vi "Measurement Logic.vi"(8 "error in":errorcluster, 11 "Measurement Configuration":T2) -> (0 "error out":errorcluster, 3 "Measurement Results":T1 {"Load Regulation (mV/mA)" format="%#.5g"})   [LabVIEW 2020, in "Load Regulation.lvlib"]
uses:
  Load Regulation.lvlib
  Reusables/Stimulus And Measure.ctl
  Reusables/Load Output Function.ctl
  Reusables/Prepare Fn Configurations.ctl
  Reusables/Advanced Settings.ctl
  26cf059d-6099-420a-9488-44e269848c92.vi
  TestResults.ctl
  TestInputs.ctl
  Measurement Results.ctl
  Measurement Configuration.ctl
panel:
  out "Load Regulation":cluster{"Iload (mA)":dbl[], "Vout (V)":dbl[]}(graph)
  out "Load Regulation (%)":dbl format="%#.3g"
  out "Load Regulation (mV/mA)":dbl format="%#.3g"
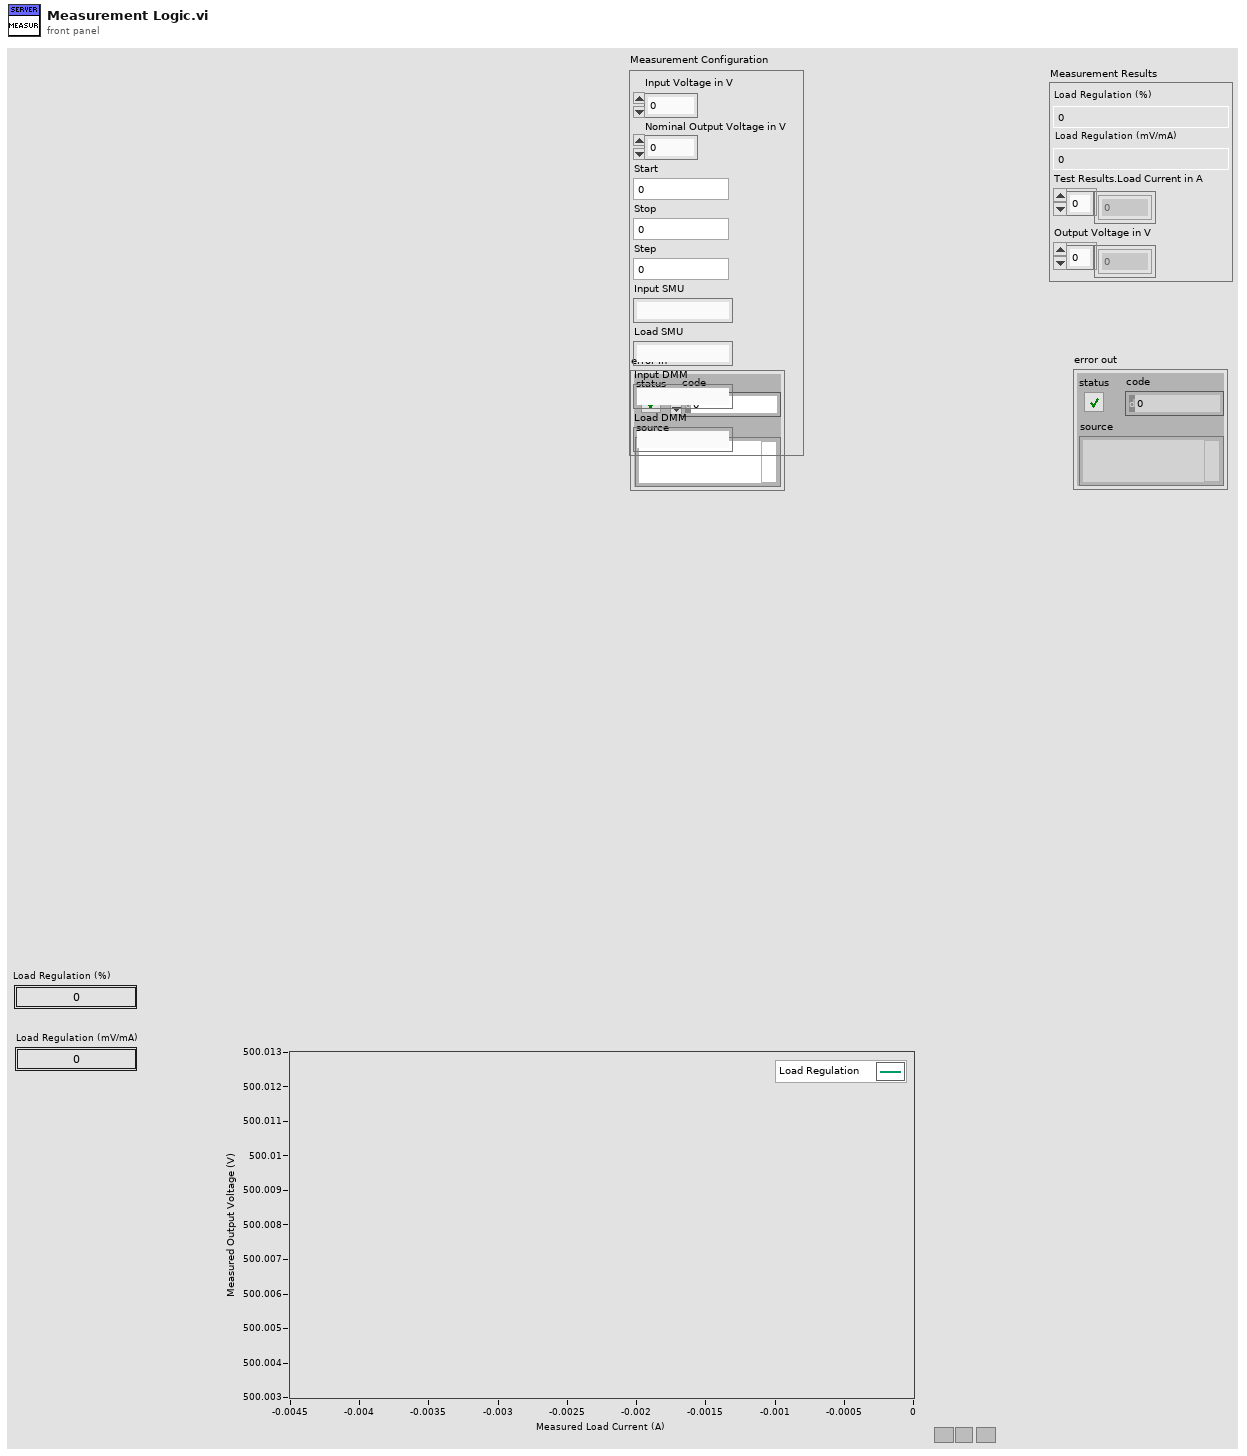
[diagram p1: front panel]
types:
  T1 = typedef "Load Regulation.lvlib/Measurement Results.ctl" = cluster{"Load Regulation (%)":dbl, "Load Regulation (mV/mA)":dbl, "Test Results.Load Current in A":dbl[], "Output Voltage in V":dbl[]}
  T2 = typedef "Load Regulation.lvlib/Measurement Configuration.ctl" = cluster{"Input Voltage in V":dbl, "Nominal Output Voltage in V":dbl, "Start":dbl, "Stop":dbl, "Step":dbl, "Input SMU":string, "Load SMU":string, "Input DMM":string, "Load DMM":string}
  T3 = typedef "Load Regulation.lvlib/TestInputs.ctl" = cluster{"Input Voltage in V":dbl, "Load Current in A":dbl[], "Nominal Output Voltage in V":dbl, "Advance Setting":T4}
  T4 = typedef "Advanced Settings.ctl" = cluster{"Prepare":T5, "Stimulus And Measure":T7}
  T5 = typedef "Prepare Fn Configurations.ctl" = cluster{"Load SMU Output Function":T6}
  T6 = typedef "Load Output Function.ctl" = enum16{"VoltageSource", "CurrentSource"}
  T7 = typedef "Stimulus And Measure.ctl" = cluster{"Loop Delay in milliSecond":u32}
  T8 = typedef "Load Regulation.lvlib/TestResults.ctl" = cluster{"Input Voltage in V":dbl[], "Input Current in A":dbl[], "Output Voltage in V":dbl[], "Load Current in A":dbl[], "Load Regulation in mV/mA":dbl, "Load Regulation in %":dbl}
  T9 = cluster{"Test Inputs":T3, "Test Results":T8, "Test Results[][]":string[][], "Input SMU":refnum<k15>, "Input DMM":refnum<k15>, "Load DMM":refnum<k15>, "Load SMU":refnum<k15>}
  T10 = cluster{"Load Current in A":dbl[], "Output Voltage in V":dbl[]}
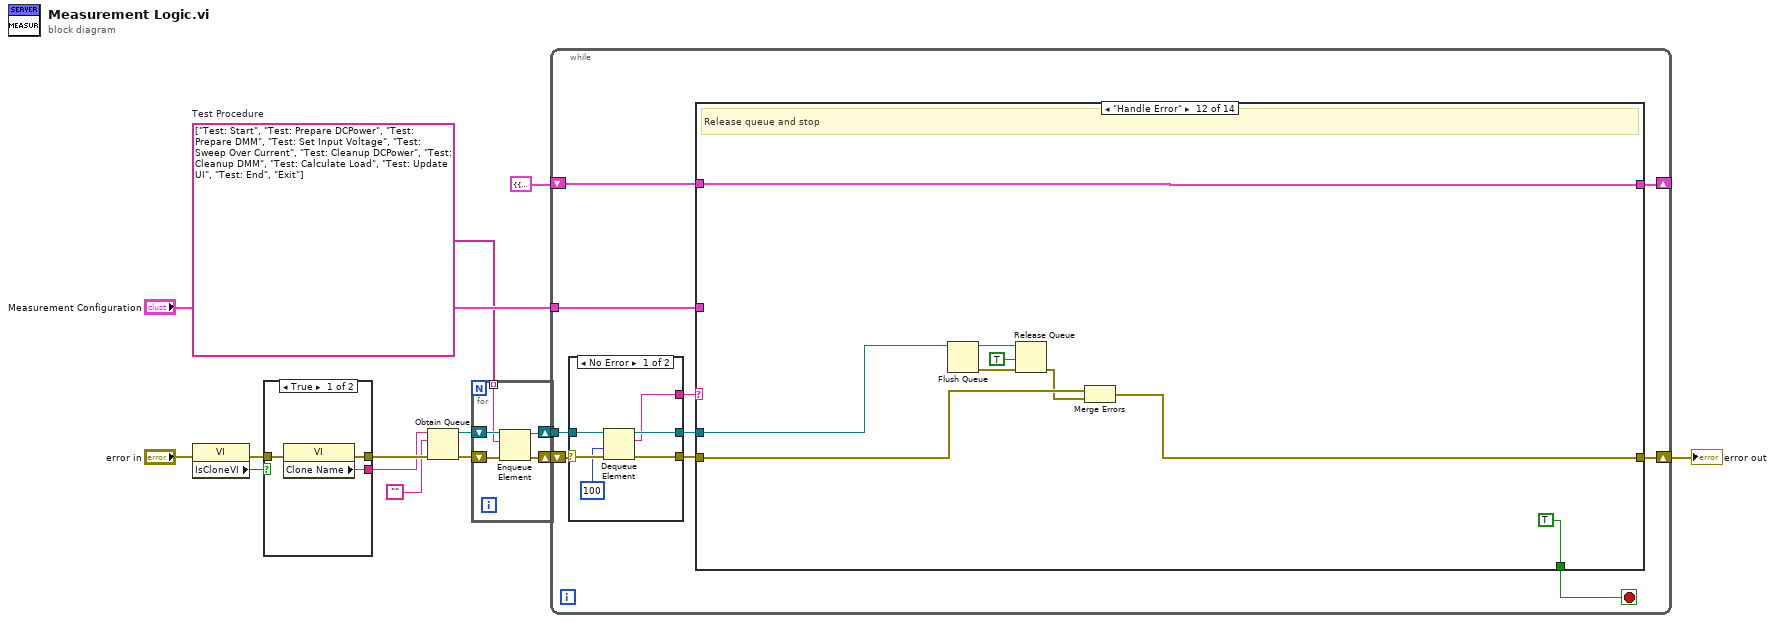
[diagram p0: block diagram]
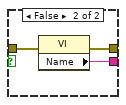
[diagram p2: hidden frame]
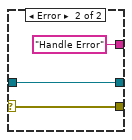
[diagram p3: hidden frame]
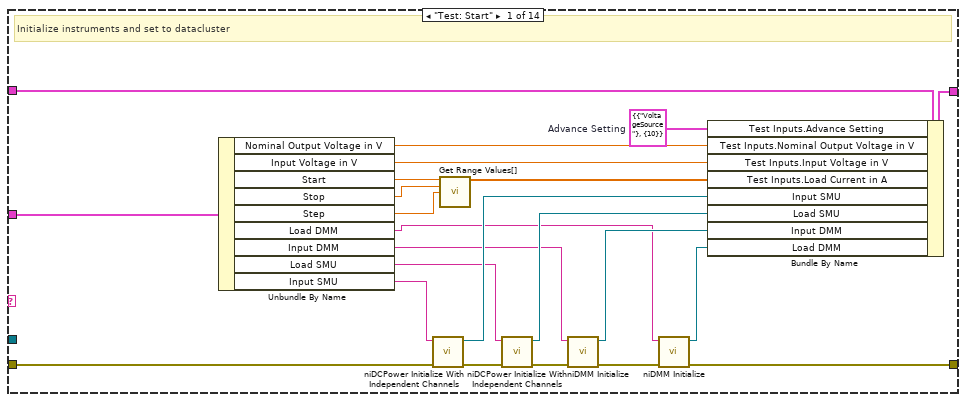
[diagram p4: hidden frame]
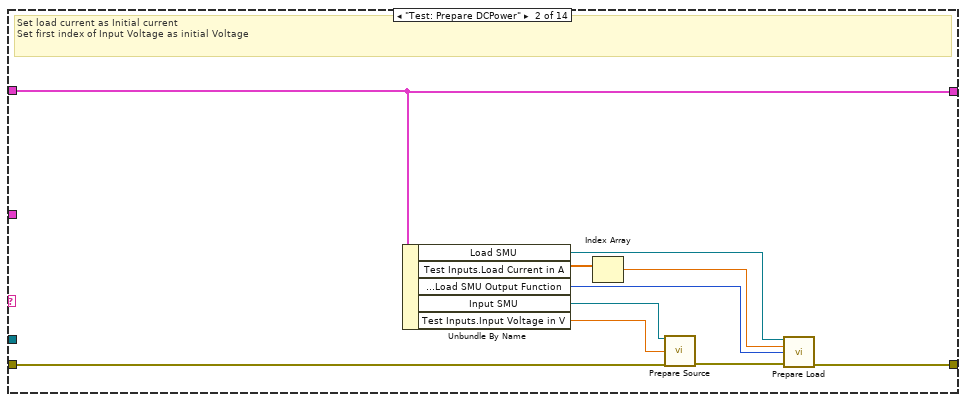
[diagram p5: hidden frame]
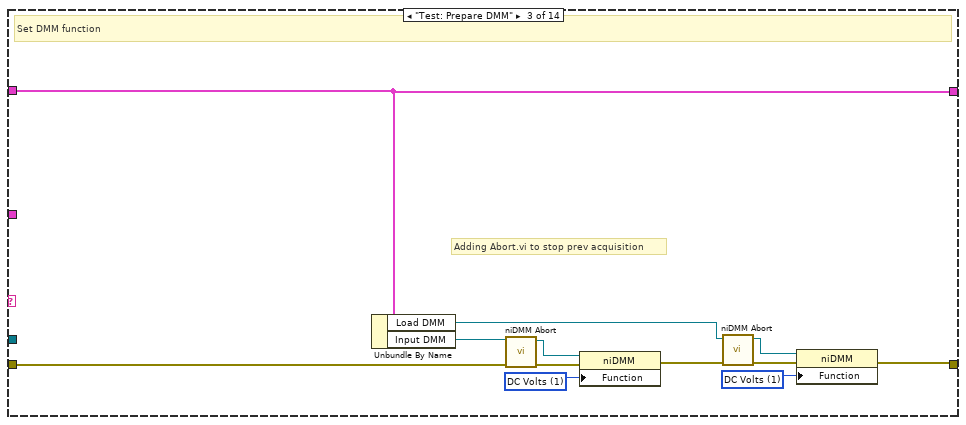
[diagram p6: hidden frame]
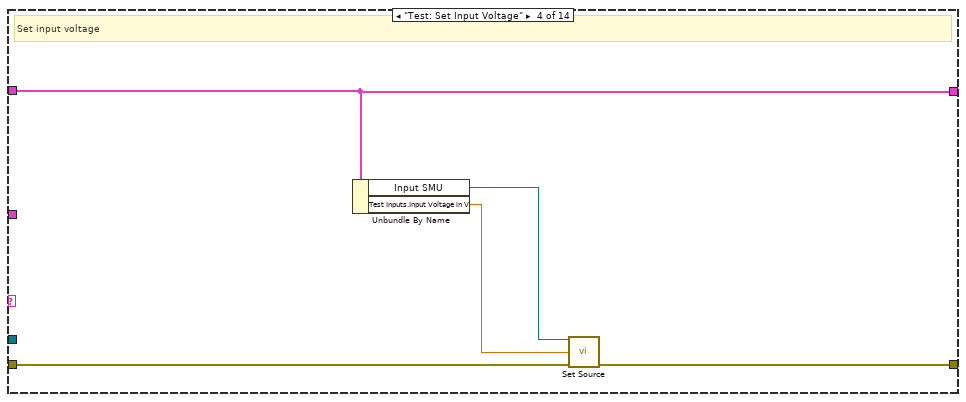
[diagram p7: hidden frame]
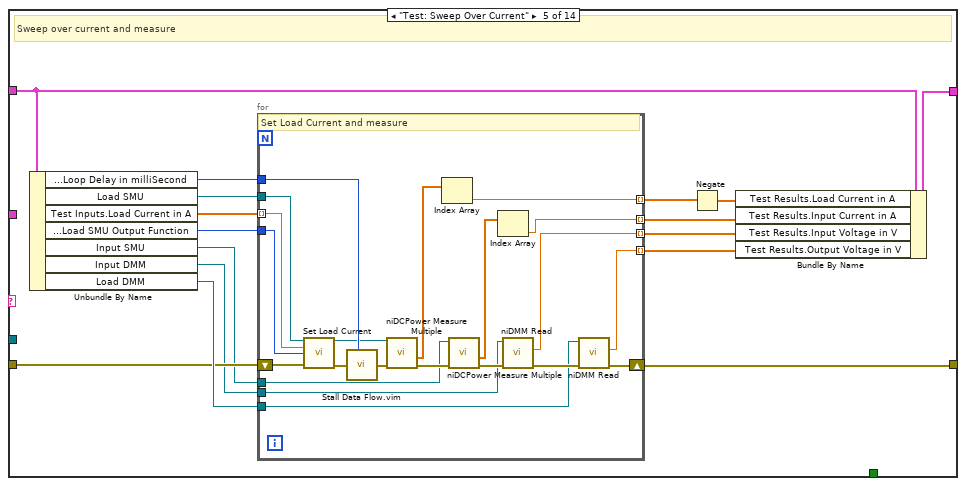
[diagram p8: hidden frame]
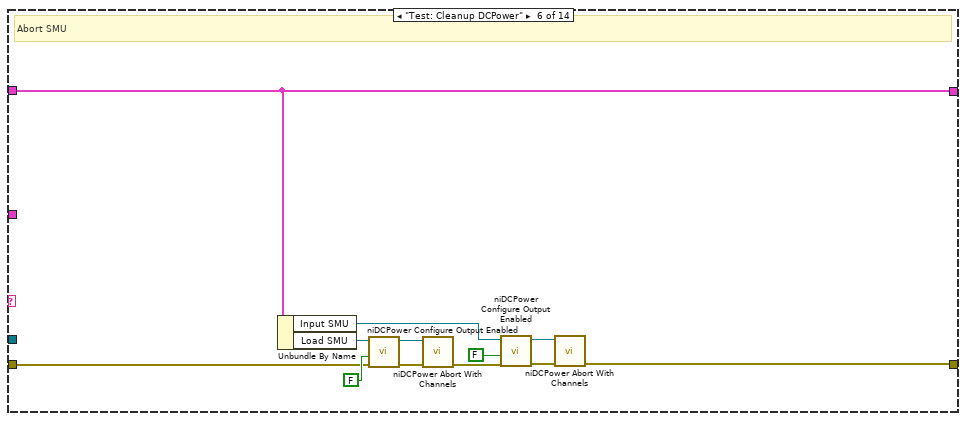
[diagram p9: hidden frame]
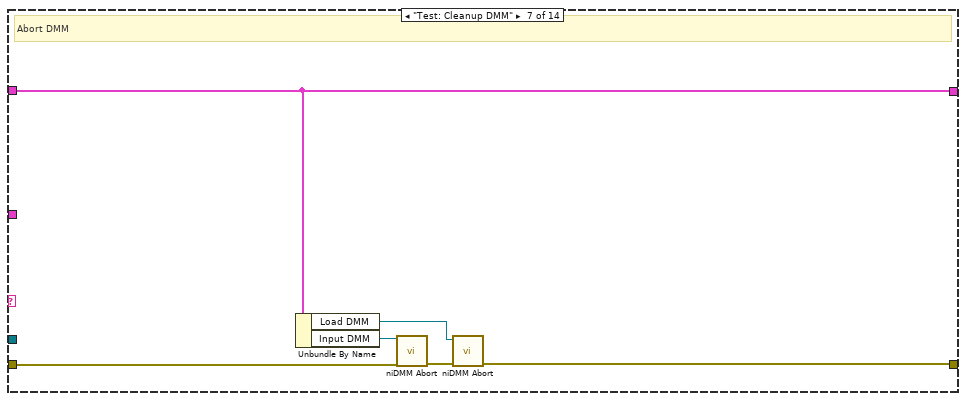
[diagram p10: hidden frame]
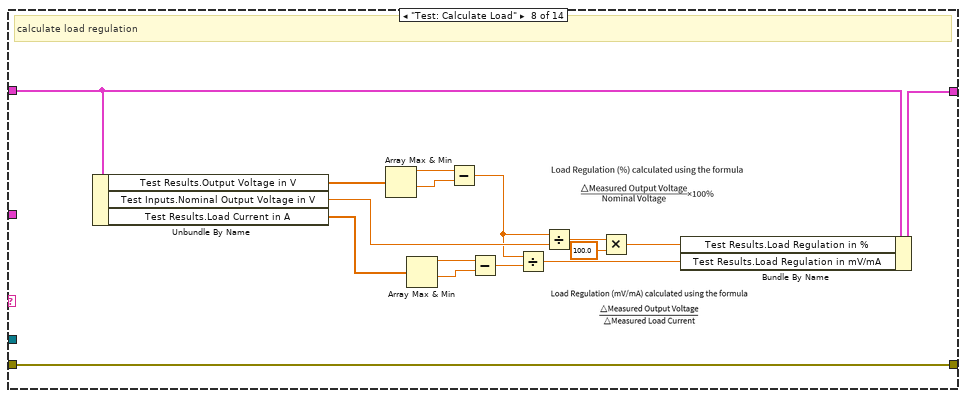
[diagram p11: hidden frame]
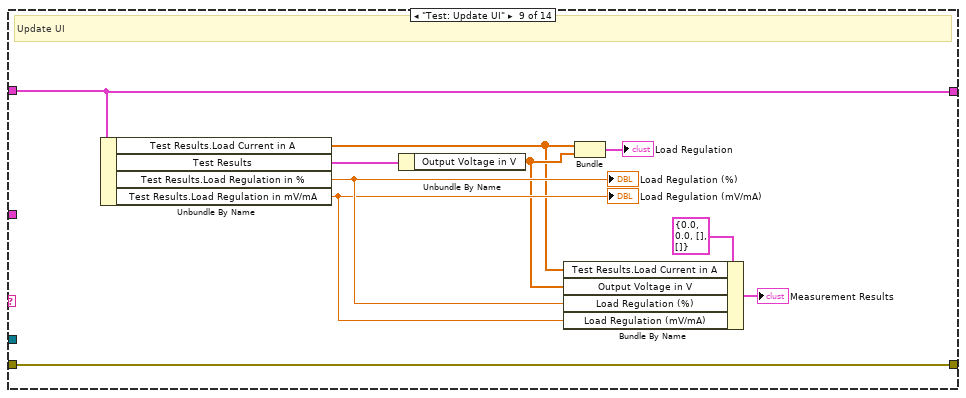
[diagram p12: hidden frame]
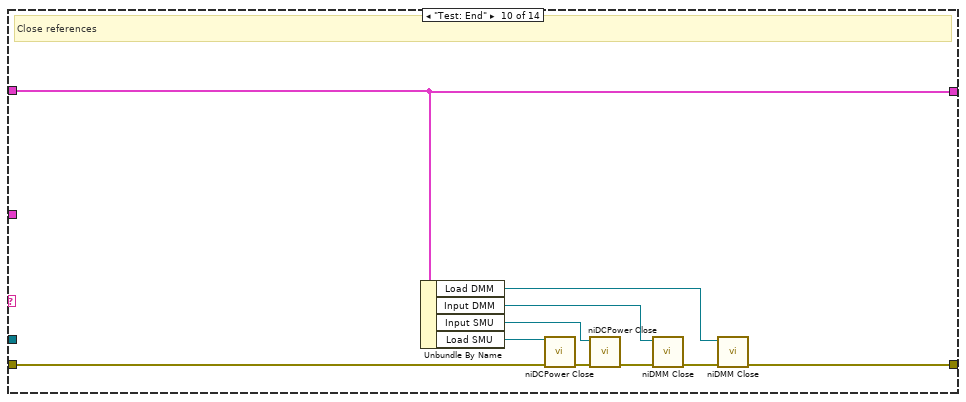
[diagram p13: hidden frame]
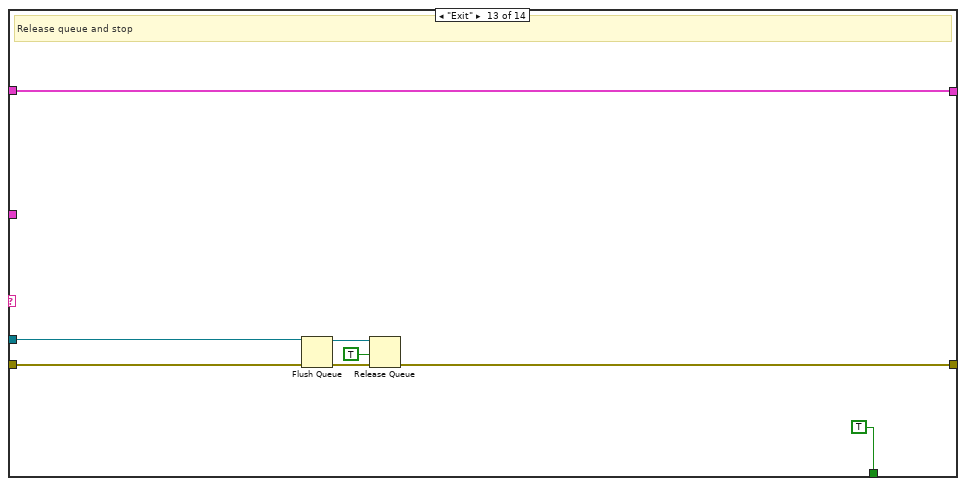
[diagram p15: hidden frame]
diagram:
  w2 = string[] ["Test: Start", "Test: Prepare DCPower", "Test: Prepare DMM", "Test: Set Input Voltage", "Test: Sweep Over Current", "Test: Cleanup DCPower", "Test: Cleanup DMM", "Test: Calculate Load", "Test: Update UI", "Test: End", "Exit"]  # Test Procedure
  n1 = property class="VI"(error in="error in") -> (error out=w7:errorcluster, "IsCloneVI"=w8:bool)  [unwired: 1 in, 1 out]
  n2 = case shown="True" w8 {
    tunnel: [w17 w20] -> w13
    tunnel: [w16 w19] -> w12
    tunnel: w7 -> [w15 w18]
    frame True {
      n3 = property class="VI"(error in=w15) -> (error out=w17:errorcluster, "Clone Name"=w16:string)  [unwired: 1 in, 1 out]
    }
    frame False {
      n4 = property class="VI"(error in=w18) -> (error out=w20:errorcluster, "Name"=w19:string)  [unwired: 1 in, 1 out]
    }
  }
  n5 = Obtain Queue(name (unnamed)=w12, element data type="", error in (no error)=w13) -> (queue out=w10:refnum<queue>, error out=w11:errorcluster)  [unwired: 2 in, 1 out]
  n6 = for {
    shift-right: [w22] -> w5
    shift-left: w11 -> [w25]
    shift-right: [w23] -> w6
    shift-left: w10 -> [w24]
    tunnel: w2 -> [w21] mode=indexing
    n7 = Enqueue Element(queue=w24, element=w21, error in (no error)=w25) -> (queue out=w23:refnum<queue>, error out=w22:errorcluster)  [unwired: 1 in, 1 out]
  }
  n8 = while {
    tunnel: w6 -> [w30]
    shift-right: [w35] -> w1
    shift-left: w5 -> [w31]
    shift-right: [w33] -> _
    shift-left: T9 {"Test Inputs"={"Input Voltage in V"=0.0, "Load Current in A"=[], "Nominal Output Voltage in V"=0.0, "Advance Setting"={"Prepare"={"Load SMU Output Function"=enum."VoltageSource"}, "Stimulus And Measure"={"Loop Delay in milliSecond"=1}}}, "Test Results"={"Input Voltage in V"=[], "Input Current in A"=[], "Output Voltage in V"=[], "Load Current in A"=[], "Load Regulation in mV/mA"=0.0, "Load Regulation in %"=0.0}, "Test Results[][]"=[], "Input SMU"="", "Input DMM"="", "Load DMM"="", "Load SMU"=""} -> [w34]
    tunnel: "Measurement Configuration" -> [w26]
    stop <- w32 stop-if-true
    n9 = case shown="No Error" w31 {
      selector: w31 -> [w41 w44]
      tunnel: [w40 w44] -> w27
      tunnel: w30 -> [w39 w43]
      tunnel: [w38 w43] -> w28
      tunnel: [w37 "Handle Error"] -> w29
      frame No Error {
        n10 = Dequeue Element(queue=w39, timeout in ms (-1)=100, error in (no error)=w41) -> (queue out=w38:refnum<queue>, element=w37:string, error out=w40:errorcluster)  [unwired: 1 out]
      }
      frame Error {
      }
    }
    n11 = case shown="\"Handle Error\"" w29 {
      tunnel: w28 -> [_ _ _ _ _ _ _ _ _ _ _ w188 w197 _]
      tunnel: w27 -> [w49 w70 w78 w90 w99 w132 w144 w150 w168 w176 w187 w194 w199 w205]
      tunnel: [w62 w71 w80 w91 w102 w140 w147 w150 w168 w179 w187 w195 w198 w205] -> w35
      tunnel: w34 -> [w66 w76 w86 w94 w100 w139 w149 w151 w173 w185 w186 w196 w204 w206]
      tunnel: [w67 w76 w86 w94 w101 w139 w149 w152 w173 w185 w186 w196 w204 w206] -> w33
      tunnel: [_ _ _ _ _ _ _ _ _ _ _ TRUE TRUE _] -> w32
      tunnel: w26 -> [w45 _ _ _ _ _ _ _ _ _ _ _ _ _]
      frame "Test: Start" {
        w48 = T4 {"Prepare"={"Load SMU Output Function"=enum."VoltageSource"}, "Stimulus And Measure"={"Loop Delay in milliSecond"=10}}  # Advance Setting
        # "Initialize instruments and set to datacluster"
        n12 = Unbundle By Name(w45) -> ("Nominal Output Voltage in V"=w57:dbl, "Input Voltage in V"=w46:dbl, "Start"=w56:dbl, "Stop"=w55:dbl, "Step"=w54:dbl, "Load DMM"=w50:string, "Input DMM"=w51:string, "Load SMU"=w52:string, "Input SMU"=w53:string)
        n13 = call <instrlib>:"niDCPower Initialize With Independent Channels.vi"("error in (no error)"=w49, "resource name"=w53) -> ("error out"=w61:errorcluster, "instrument handle out"=w65:refnum<k15>)  [unwired: 8 in]
        n14 = call "Get Range Values[].vi"("Start"=w56, "Stop"=w55, "Step Size"=w54) -> ("Values[]"=w47:dbl[])  [unwired: 12 in]
        n15 = call <instrlib>:"niDCPower Initialize With Independent Channels.vi"("error in (no error)"=w61, "resource name"=w52) -> ("error out"=w60:errorcluster, "instrument handle out"=w58:refnum<k15>)  [unwired: 8 in]
        n16 = call <instrlib>:"niDMM Initialize.vi"("error in (no error)"=w60, "Instrument Descriptor"=w51) -> ("error out"=w63:errorcluster, "instrument handle out"=w59:refnum<k15>)  [unwired: 8 in]
        n17 = call <instrlib>:"niDMM Initialize.vi"("error in (no error)"=w63, "Instrument Descriptor"=w50) -> ("error out"=w62:errorcluster, "instrument handle out"=w64:refnum<k15>)  [unwired: 8 in]
        n18 = Bundle By Name(cluster=w66, "Test Inputs.Advance Setting"=w48, "Test Inputs.Nominal Output Voltage in V"=w57, "Test Inputs.Input Voltage in V"=w46, "Test Inputs.Load Current in A"=w47, "Input SMU"=w65, "Load SMU"=w58, "Input DMM"=w59, "Load DMM"=w64) -> (w67:T9)
      }
      frame "Test: Prepare DCPower" {
        # "Set load current as Initial current\nSet first index of Input Voltage as initial Voltage"
        n19 = Unbundle By Name(w76) -> ("Load SMU"=w74:refnum<k15>, "Test Inputs.Load Current in A"=w73:dbl[], "Test Inputs.Advance Setting.Prepare.Load SMU Output Function"=w68:T6, "Input SMU"=w75:refnum<k15>, "Test Inputs.Input Voltage in V"=w77:dbl)
        n20 = Index Array(array=w73) -> (element=w69:dbl)  [unwired: 1 in]
        n21 = call "Prepare Source.vi"("instrument handle"=w75, "Initial Voltage Level (V)"=w77, "error in (no error)"=w70) -> ("error out"=w72:errorcluster)  [unwired: 12 in]
        n22 = call "Prepare Load.vi"("instrument handle"=w74, "Load Current Level (A)"=w69, "Load Output Function"=w68, "error in (no error)"=w72) -> ("error out"=w71:errorcluster)  [unwired: 11 in]
      }
      frame "Test: Prepare DMM" {
        w82 = 1 items=["DC Volts"=1, "AC Volts"=2, "DC Current"=3, "AC Current"=4, "2-Wire Resistance"=5, "4-Wire Resistance"=101, "Frequency"=104, "Period"=105, "AC Volts DC Coupled"=1001, "Diode"=1002, "Waveform Voltage"=1003, "Waveform Current"=1004, "Capacitance"=1005, "Inductance"=1006, "Temperature"=108] ("Configuration:Function")
        w89 = 1 items=["DC Volts"=1, "AC Volts"=2, "DC Current"=3, "AC Current"=4, "2-Wire Resistance"=5, "4-Wire Resistance"=101, "Frequency"=104, "Period"=105, "AC Volts DC Coupled"=1001, "Diode"=1002, "Waveform Voltage"=1003, "Waveform Current"=1004, "Capacitance"=1005, "Inductance"=1006, "Temperature"=108] ("Configuration:Function")
        # "Adding Abort.vi to stop prev acquisition"
        # "Set DMM function"
        n23 = Unbundle By Name(w86) -> ("Load DMM"=w79:refnum<k15>, "Input DMM"=w85:refnum<k15>)
        n24 = call <instrlib>:"niDMM Abort.vi"("error in (no error)"=w78, "instrument handle"=w85) -> ("error out"=w88:errorcluster, "instrument handle out"=w87:refnum<k15>)  [unwired: 8 in]
        n25 = property class="niDMM"(reference=w87, error in=w88, "Function"=w89) -> (error out=w81:errorcluster)  [unwired: 1 out]
        n26 = call <instrlib>:"niDMM Abort.vi"("error in (no error)"=w81, "instrument handle"=w79) -> ("error out"=w83:errorcluster, "instrument handle out"=w84:refnum<k15>)  [unwired: 8 in]
        n27 = property class="niDMM"(reference=w84, error in=w83, "Function"=w82) -> (error out=w80:errorcluster)  [unwired: 1 out]
      }
      frame "Test: Set Input Voltage" {
        # "Set input voltage"
        n28 = Unbundle By Name(w94) -> ("Input SMU"=w93:refnum<k15>, "Test Inputs.Input Voltage in V"=w92:dbl)
        n29 = call "Set Source.vi"("instrument handle in"=w93, "Vin in V"=w92, "error in (no error)"=w90) -> ("error out"=w91:errorcluster)  [unwired: 11 in, 1 out]
      }
      frame "Test: Sweep Over Current" {
        # "Sweep over current and measure"
        n30 = Unbundle By Name(w100) -> ("Test Inputs.Advance Setting.Stimulus And Measure.Loop Delay in milliSecond"=w108:u32, "Load SMU"=w110:refnum<k15>, "Test Inputs.Load Current in A"=w109:dbl[], "Test Inputs.Advance Setting.Prepare.Load SMU Output Function"=w98:T6, "Input SMU"=w95:refnum<k15>, "Input DMM"=w96:refnum<k15>, "Load DMM"=w107:refnum<k15>)
        n31 = for {
          tunnel: w110 -> [w130]
          tunnel: w109 -> [w113] mode=indexing
          tunnel: w108 -> [w128]
          tunnel: w96 -> [w121]
          tunnel: w107 -> [w120]
          tunnel: [w114] -> w106 mode=indexing
          tunnel: [w115] -> w105 mode=indexing
          tunnel: [w119] -> w104 mode=indexing
          tunnel: [w118] -> w103 mode=indexing
          shift-right: [w117] -> w102
          shift-left: w99 -> [w131]
          tunnel: w98 -> [w112]
          tunnel: w95 -> [w111]
          # "Set Load Current and measure"
          n32 = call "Set Load Current.vi"("instrument handle in"=w130, "current level"=w113, "OutputFunction"=w112, "error in (no error)"=w131) -> ("instrument handle out"=w116:refnum<k15>, "error out"=w129:errorcluster)  [unwired: 10 in]
          n33 = call "Stall Data Flow.vim"("value in"=w129, "milliseconds to wait"=w128) -> ("value out"=w122:errorcluster)  [unwired: 1 out]
          n34 = call <instrlib>:"niDCPower Measure Multiple.vi"("error in (no error)"=w122, "instrument handle"=w116) -> ("error out"=w124:errorcluster, "current measurements"=w127:dbl[])  [unwired: 6 in, 2 out]
          n35 = Index Array(array=w127) -> (element=w115:dbl)  [unwired: 1 in]
          n36 = call <instrlib>:"niDCPower Measure Multiple.vi"("error in (no error)"=w124, "instrument handle"=w111) -> ("error out"=w123:errorcluster, "current measurements"=w125:dbl[])  [unwired: 6 in, 2 out]
          n37 = Index Array(array=w125) -> (element=w114:dbl)  [unwired: 1 in]
          n38 = call <instrlib>:"niDMM Read.vi"("error in (no error)"=w123, "instrument handle"=w121) -> ("error out"=w126:errorcluster, "Measurement"=w119:dbl)  [unwired: 7 in, 1 out]
          n39 = call <instrlib>:"niDMM Read.vi"("error in (no error)"=w126, "instrument handle"=w120) -> ("error out"=w117:errorcluster, "Measurement"=w118:dbl)  [unwired: 7 in, 1 out]
        }
        n40 = Negate(x=w105) -> (-x=w97:dbl[])
        n41 = Bundle By Name(cluster=w100, "Test Results.Load Current in A"=w97, "Test Results.Input Current in A"=w106, "Test Results.Input Voltage in V"=w104, "Test Results.Output Voltage in V"=w103) -> (w101:T9)
      }
      frame "Test: Cleanup DCPower" {
        # "Abort SMU"
        n42 = Unbundle By Name(w139) -> ("Input SMU"=w138:refnum<k15>, "Load SMU"=w133:refnum<k15>)
        n43 = call <instrlib>:"niDCPower Configure Output Enabled.vi"("error in (no error)"=w132, "output enabled"=FALSE, "instrument handle"=w133) -> ("error out"=w134:errorcluster, "instrument handle out"=w137:refnum<k15>)  [unwired: 7 in]
        n44 = call <instrlib>:"niDCPower Abort With Channels.vi"("error in (no error)"=w134, "instrument handle"=w137) -> ("error out"=w135:errorcluster)  [unwired: 8 in, 1 out]
        n45 = call <instrlib>:"niDCPower Configure Output Enabled.vi"("error in (no error)"=w135, "output enabled"=FALSE, "instrument handle"=w138) -> ("error out"=w142:errorcluster, "instrument handle out"=w141:refnum<k15>)  [unwired: 7 in]
        n46 = call <instrlib>:"niDCPower Abort With Channels.vi"("error in (no error)"=w142, "instrument handle"=w141) -> ("error out"=w140:errorcluster)  [unwired: 8 in, 1 out]
      }
      frame "Test: Cleanup DMM" {
        # "Abort DMM"
        n47 = Unbundle By Name(w149) -> ("Load DMM"=w146:refnum<k15>, "Input DMM"=w145:refnum<k15>)
        n48 = call <instrlib>:"niDMM Abort.vi"("error in (no error)"=w144, "instrument handle"=w145) -> ("error out"=w148:errorcluster)  [unwired: 8 in, 1 out]
        n49 = call <instrlib>:"niDMM Abort.vi"("error in (no error)"=w148, "instrument handle"=w146) -> ("error out"=w147:errorcluster)  [unwired: 8 in, 1 out]
      }
      frame "Test: Calculate Load" {
        # "calculate load regulation"
        n50 = Unbundle By Name(w151) -> ("Test Results.Output Voltage in V"=w162:dbl[], "Test Inputs.Nominal Output Voltage in V"=w160:dbl, "Test Results.Load Current in A"=w157:dbl[])
        n51 = Array Max & Min(array=w162) -> (max value=w165:dbl, min value=w161:dbl)  [unwired: 2 out]
        n52 = Array Max & Min(array=w157) -> (max value=w158:dbl, min value=w159:dbl)  [unwired: 2 out]
        n53 = Subtract(x=w165, y=w161) -> (x-y=w156:dbl)
        n54 = Subtract(x=w158, y=w159) -> (x-y=w155:dbl)
        n55 = Divide(x=w156, y=w155) -> (x/y=w154:dbl)
        n56 = Divide(x=w156, y=w160) -> (x/y=w164:dbl)
        n57 = Multiply(x=w164, y=100.0) -> (x*y=w163:dbl)
        n58 = Bundle By Name(cluster=w151, "Test Results.Load Regulation in %"=w163, "Test Results.Load Regulation in mV/mA"=w154) -> (w152:T9)
      }
      frame "Test: Update UI" {
        # "Update UI"
        n59 = Unbundle By Name(w173) -> ("Test Results.Load Current in A"=w169:dbl[], "Test Results"=w175:T8, "Test Results.Load Regulation in %"=w172:dbl, "Test Results.Load Regulation in mV/mA"=w171:dbl)
        "Load Regulation (%)" <- w172
        "Load Regulation (mV/mA)" <- w171
        n60 = Unbundle By Name(w175) -> ("Output Voltage in V"=w170:dbl[])
        n61 = Bundle By Name(cluster=T1 {"Load Regulation (%)"=0.0, "Load Regulation (mV/mA)"=0.0, "Test Results.Load Current in A"=[], "Output Voltage in V"=[]} ("Measurement Results"), "Test Results.Load Current in A"=w169, "Output Voltage in V"=w170, "Load Regulation (%)"=w172, "Load Regulation (mV/mA)"=w171) -> (→"Measurement Results":T1)
        n62 = Bundle("Load Current in A"=w169, "Output Voltage in V"=w170) -> (→"Load Regulation":T10)  [unwired: 1 in]
      }
      frame "Test: End" {
        # "Close references"
        n63 = Unbundle By Name(w185) -> ("Load DMM"=w180:refnum<k15>, "Input DMM"=w181:refnum<k15>, "Input SMU"=w184:refnum<k15>, "Load SMU"=w178:refnum<k15>)
        n64 = call <instrlib>:"niDCPower Close.vi"("error in (no error)"=w176, "instrument handle"=w178) -> ("error out"=w177:errorcluster)  [unwired: 9 in]
        n65 = call <instrlib>:"niDCPower Close.vi"("error in (no error)"=w177, "instrument handle"=w184) -> ("error out"=w183:errorcluster)  [unwired: 9 in]
        n66 = call <instrlib>:"niDMM Close.vi"("error in (no error)"=w183, "instrument handle"=w181) -> ("error out"=w182:errorcluster)  [unwired: 9 in]
        n67 = call <instrlib>:"niDMM Close.vi"("error in (no error)"=w182, "instrument handle"=w180) -> ("error out"=w179:errorcluster)  [unwired: 9 in]
      }
      frame "----Misc------" {
      }
      frame "Handle Error" {
        # "Release queue and stop"
        n68 = Flush Queue(queue=w188) -> (queue out=w192:refnum<queue>, error out=w191:errorcluster)  [unwired: 1 in, 1 out]
        n69 = Release Queue(queue=w192, force destroy? (F)=TRUE, error in (no error)=w191) -> (error out=w189:errorcluster)  [unwired: 2 out]
        n70 = Merge Errors(w194, w189) -> (w195:errorcluster)
      }
      frame "Exit" {
        # "Release queue and stop"
        n71 = Flush Queue(queue=w197, error in (no error)=w199) -> (queue out=w202:refnum<queue>, error out=w201:errorcluster)  [unwired: 1 out]
        n72 = Release Queue(queue=w202, force destroy? (F)=TRUE, error in (no error)=w201) -> (error out=w198:errorcluster)  [unwired: 2 out]
      }
      frame "", Default {
        # "Do nothing"
      }
    }
  }
  "error out" <- w1
